vi "gRPC Port FGV.vi"(7 "Op (Get)":enum16{"Get", "Set"}(ring), 11 "Listening Port in":i32) -> (3 "Listening Port out":i32)   [LabVIEW 2025]
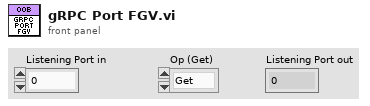
[diagram p1: front panel]
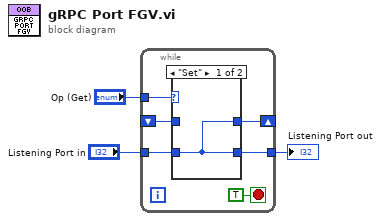
[diagram p0: block diagram]
diagram:
  n1 = while {
    tunnel: "Op (Get)" -> [w8]
    shift-right: [w7] -> _
    shift-left: _ -> [w6]
    tunnel: "Listening Port in" -> [w5]
    tunnel: [w4] -> w1
    stop <- TRUE stop-if-true
    n2 = case shown="\"Set\"" w8 {
      tunnel: [w10 w11] -> w7
      tunnel: w6 -> [_ w11]
      tunnel: w5 -> [w10 _]
      tunnel: [w10 w11] -> w4
      frame "Set" {
      }
      frame "Get" {
      }
    }
  }
  "Listening Port out" <- w1
